vi "Token Key.vi"(8 "Error In":errorcluster, 11 "Token":refnum<class "Token.lvclass">) -> (0 "Error Out":errorcluster, 3 "Key":string)   [LabVIEW 2018, in "Toolkit.lvlib" / "Parser.lvclass"]
uses:
  Parser.lvclass
  Tokens/Token/Token.lvclass
  Tokens/Keyable/Keyable.lvclass
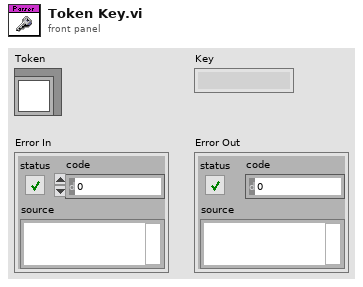
[diagram p1: front panel]
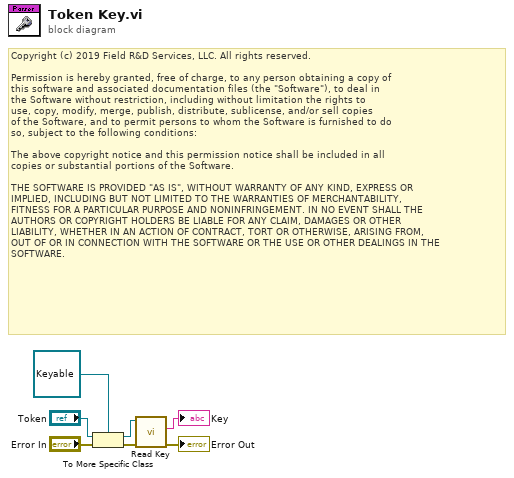
[diagram p0: block diagram]
diagram:
  # "Copyright (c) 2019 Field R&D Services, LLC. All rights reserved.\n\nPermission is hereby granted, free of charge, to any person obtaining a copy of\nthis software and associated documentation files (the \"Software\"), to deal in\nthe Software without restriction, including without limitation the rights to\nuse, copy, modify, merge, publish, distribute, sublicense, and/or sell copies\nof the Software, and to permit persons to whom the Software is furnished to do\nso, subject to the following conditions:\n\nThe above copyright notice and this permission notice shall be included in all\ncopies or substantial portions of the Software.\n\nTHE SOFTWARE IS PROVIDED \"AS IS\", WITHOUT WARRANTY OF ANY KIND, EXPRESS OR\nIMPLIED, INCLUDING BUT NOT LIMITED TO THE WARRANTIES OF MERCHANTABILITY,\nFITNESS FOR A PARTICULAR PURPOSE AND NONINFRINGEMENT. IN NO EVENT SHALL THE\nAUTHORS OR COPYRIGHT HOLDERS BE LIABLE FOR ANY CLAIM, DAMAGES OR OTHER\nLIABILITY, WHETHER IN AN ACTION OF CONTRACT, TORT OR OTHERWISE, ARISING FROM,\nOUT OF OR IN CONNECTION WITH THE SOFTWARE OR THE USE OR OTHER DEALINGS IN THE\nSOFTWARE."
  n1 = To More Specific Class(target class=refnum<class "Keyable.lvclass"> refnum ("Toolkit.lvlib:Tokens.lvlib:Keyable.lvclass"), reference="Token", error in="Error In") -> (specific class reference=w4:refnum<class "Keyable.lvclass">, error out=w3:errorcluster)
  n2 = call-dynamic "Read Key.vi"("Error In"=w3, "Keyable In"=w4) -> ("Error Out"=→"Error Out":errorcluster, "Key"=→"Key":string)  [unwired: 7 in, 1 out]
